vi "solar_visa VISA Query.vi"(4 "VISA Read Timeout (0 = Ignore)":u32, 6 "ms Read Wait (0)":u32, 8 "error in (no error)":errorcluster, 9 "Bytes Expected (0 = No Read)":u32, 10 "Write (\"\" = No Write)":string, 11 "VISA Resource in":refnum<visa-resource-name>) -> (0 "error out":errorcluster, 1 "Bytes Recieved":u32, 2 "Read":string, 3 "VISA Resource out":refnum<visa-resource-name>)   [LabVIEW 2018]
doc: "This queries data from the VISA session. Set <b>ms Read Wait</b> to wait in milliseconds between writing and reading.\nIf <b>Write</b> is empty this does not write data to the VISA session.\nIf <b>Bytes Expected</b> is 0 this does not read data from the VISA session.\nIf <b>VISA Read Timeout</b> is greater than 0 this temporarily sets the VISA timeout for this query only then resets the timeout.\nIf <b>Simulate</b> is true this returns the <b>Simulate Read</b> data."
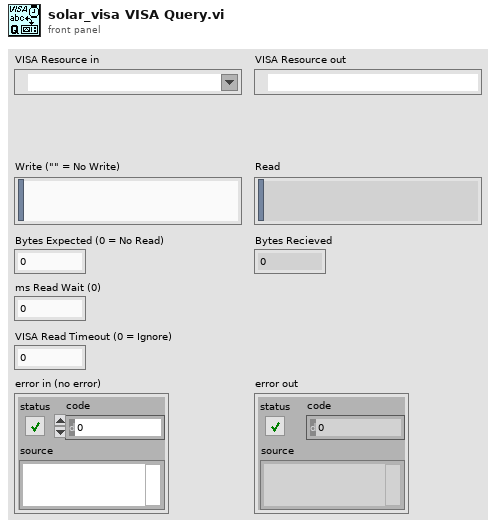
[diagram p1: front panel]
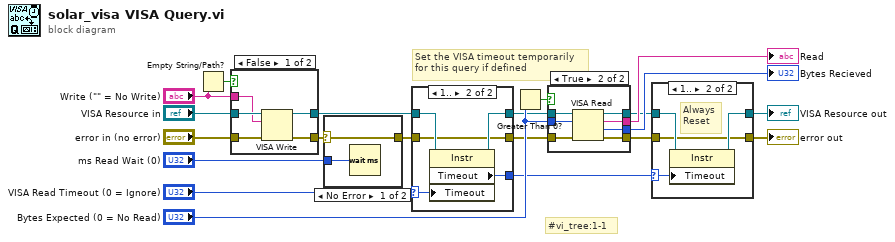
[diagram p0: block diagram]
diagram:
  # "#vi_tree:1-1"
  # "Set the VISA timeout temporarily\nfor this query if defined"
  n1 = Empty String/Path?(string/path="Write (\"\" = No Write)") -> (empty?=w10:bool)
  n2 = case shown="False" w10 {
    tunnel: "error in (no error)" -> [w25 w27]
    tunnel: "VISA Resource in" -> [w24 w26]
    tunnel: "Write (\"\" = No Write)" -> [w22 _]
    tunnel: [w23 w27] -> w8
    tunnel: [w21 w26] -> w7
    frame False {
      n3 = VISA Write(VISA resource name=w24, write buffer=w22, error in (no error)=w25) -> (VISA resource name out=w21:refnum<visa-resource-name>, error out=w23:errorcluster)  [unwired: 1 out]
    }
    frame True {
    }
  }
  n4 = case shown="No Error" w8 {
    tunnel: "ms Read Wait (0)" -> [w29 _]
    tunnel: [w28 w30] -> w9
    selector: w8 -> [w28 w30]
    frame No Error {
      n5 = Wait (ms)(milliseconds to wait=w29) -> ()  [unwired: 1 out]
    }
    frame Error {
      # "Do not\nwait"
    }
  }
  n6 = case shown="1.." "VISA Read Timeout (0 = Ignore)" {
    selector: "VISA Read Timeout (0 = Ignore)" -> [_ w36]
    tunnel: [w31 w33] -> w5
    tunnel: [w32 w37] -> w6
    tunnel: w9 -> [w31 w33]
    tunnel: w7 -> [w32 w35]
    tunnel: [_ w34] -> w1
    frame 0 {
    }
    frame 1.. {
      n7 = property class="Instr"(reference=w35, "Timeout"=w36) -> (reference out=w37:refnum<visa-resource-name>, "Timeout"=w34:u32)  [unwired: 1 in, 1 out]
    }
  }
  n8 = Greater Than 0?(x="Bytes Expected (0 = No Read)") -> (x > 0?=w4:bool)
  n9 = case shown="True" w4 {
    tunnel: w6 -> [w39 w46]
    tunnel: [w39 w45] -> w3
    tunnel: w5 -> [w38 w44]
    tunnel: [w38 w43] -> w2
    tunnel: "Bytes Expected (0 = No Read)" -> [_ w42]
    tunnel: [_ w41] -> w12
    tunnel: [_ w40] -> w11
    frame False {
    }
    frame True {
      n10 = VISA Read(VISA resource name=w46, byte count=w42, error in (no error)=w44) -> (VISA resource name out=w45:refnum<visa-resource-name>, read buffer=w41:string, return count=w40:u32, error out=w43:errorcluster)
    }
  }
  "Read" <- w12
  "Bytes Recieved" <- w11
  n11 = case shown="1.." w1 {
    selector: w1 -> [_ w51]
    tunnel: [w47 w49] -> w18
    tunnel: [w48 w52] -> w17
    tunnel: w2 -> [w47 w49]
    tunnel: w3 -> [w48 w50]
    frame 0 {
    }
    frame 1.. {
      # "Always\nReset"
      n12 = property class="Instr"(reference=w50, "Timeout"=w51) -> (reference out=w52:refnum<visa-resource-name>)  [unwired: 1 in, 1 out]
    }
  }
  "error out" <- w18
  "VISA Resource out" <- w17
